vi "fastseq_set_orders.vi"(0 "FPGA VI Reference In":T2, 1 "us per DAC":u32=1000, 2 "pulse length":u16=100, 3 "start index":u16, 4 "Enum":T1(ring)) -> (5 "FPGA VI Reference Out":T2)   [LabVIEW 2013]
uses:
  fpga-bitfile-ref.ctl
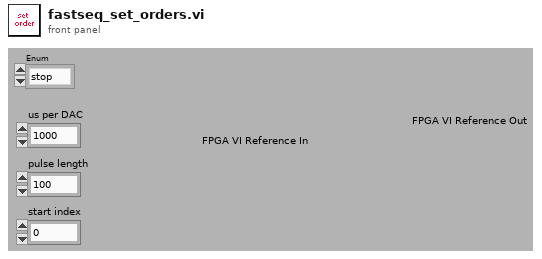
[diagram p1: front panel]
types:
  T1 = enum16{"stop", "start", "restart", "set RT", "set ramp", "set trigger length"}
  T2 = typedef "fpga-bitfile-ref.ctl" = refnum<k20>
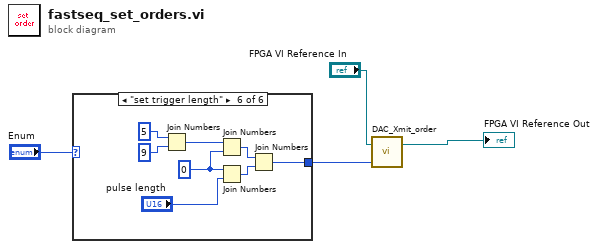
[diagram p0: block diagram]
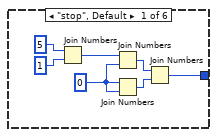
[diagram p2: hidden frame]
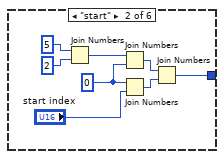
[diagram p3: hidden frame]
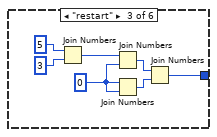
[diagram p4: hidden frame]
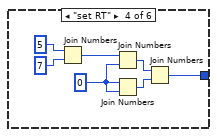
[diagram p5: hidden frame]
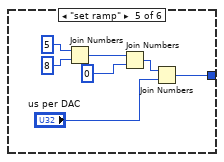
[diagram p6: hidden frame]
diagram:
  n1 = case shown="\"set trigger length\"" "Enum" {
    tunnel: [w5 w13 w21 w27 w35 w42] -> w1
    frame "stop", Default {
      w6 = u16 0 ("lo")
      n2 = Join Numbers(hi=u8 5, lo=u8 1) -> ((hi.lo)=w10:u16)
      n3 = Join Numbers(hi=w10, lo=w6) -> ((hi.lo)=w8:u32)
      n4 = Join Numbers(hi=w6, lo=w6) -> ((hi.lo)=w11:u32)
      n5 = Join Numbers(hi=w8, lo=w11) -> ((hi.lo)=w5:u64)
    }
    frame "start" {
      w14 = u16 0 ("lo")
      n6 = Join Numbers(hi=u8 5, lo=u8 2) -> ((hi.lo)=w18:u16)
      n7 = Join Numbers(hi=w18, lo=w14) -> ((hi.lo)=w16:u32)
      n8 = Join Numbers(hi=w14, lo="start index") -> ((hi.lo)=w19:u32)
      n9 = Join Numbers(hi=w16, lo=w19) -> ((hi.lo)=w13:u64)
    }
    frame "restart" {
      w20 = u16 0 ("lo")
      n10 = Join Numbers(hi=u8 5, lo=u8 3) -> ((hi.lo)=w25:u16)
      n11 = Join Numbers(hi=w25, lo=w20) -> ((hi.lo)=w23:u32)
      n12 = Join Numbers(hi=w20, lo=w20) -> ((hi.lo)=w26:u32)
      n13 = Join Numbers(hi=w23, lo=w26) -> ((hi.lo)=w21:u64)
    }
    frame "set RT" {
      w28 = u16 0 ("lo")
      n14 = Join Numbers(hi=u8 5, lo=u8 7) -> ((hi.lo)=w32:u16)
      n15 = Join Numbers(hi=w32, lo=w28) -> ((hi.lo)=w30:u32)
      n16 = Join Numbers(hi=w28, lo=w28) -> ((hi.lo)=w33:u32)
      n17 = Join Numbers(hi=w30, lo=w33) -> ((hi.lo)=w27:u64)
    }
    frame "set ramp" {
      n18 = Join Numbers(hi=u8 5, lo=u8 8) -> ((hi.lo)=w40:u16)
      n19 = Join Numbers(hi=w40, lo=u16 0) -> ((hi.lo)=w38:u32)
      n20 = Join Numbers(hi=w38, lo="us per DAC") -> ((hi.lo)=w35:u64)
    }
    frame "set trigger length" {
      w43 = u16 0 ("lo")
      n21 = Join Numbers(hi=u8 5, lo=u8 9) -> ((hi.lo)=w47:u16)
      n22 = Join Numbers(hi=w47, lo=w43) -> ((hi.lo)=w45:u32)
      n23 = Join Numbers(hi=w43, lo="pulse length") -> ((hi.lo)=w48:u32)
      n24 = Join Numbers(hi=w45, lo=w48) -> ((hi.lo)=w42:u64)
    }
  }
  n25 = call "DAC_Xmit_order.vi"("Order in"=w1, "FPGA VI Reference In"="FPGA VI Reference In") -> ("FPGA VI Reference Out"=→"FPGA VI Reference Out":T2)  [unwired: 1 out]
